vi "_Override Error.vi"(10 "Error":errorcluster) -> (2 "Override Error Msg Strategy out":refnum<class "Override Error Msg Strategy.lvclass">)   [LabVIEW 2021, in "jettl Msg Override Error.lvlib"]
uses:
  jettl Msg Override Error.lvlib
  Override Error Msg Strategy/Override Error Msg Strategy.lvclass
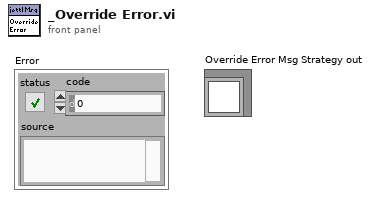
[diagram p1: front panel]
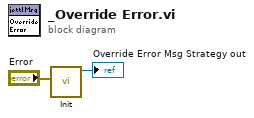
[diagram p0: block diagram]
diagram:
  n1 = call "Init.vi"("Error"="Error") -> ("Override Error Msg Strategy out"=→"Override Error Msg Strategy out":refnum<class "Override Error Msg Strategy.lvclass">)  [unwired: 10 in]
